vi "Teleop.vi"(10 "Match Info":T1={"Autonomous Elapsed Seconds"=0.0, "TeleOp Elapsed Seconds"=0.0, "Disabled Elapsed Seconds"=0.0, "Visited Autonomous"=FALSE, "Visited TeleOp"=FALSE, "Visited Disabled"=FALSE, "Autonomous Settings"={"Autonomous Style"=enum."Independent", "VI Refnum"=refnum}}, 11 "Call Context":T2) -> ()   [LabVIEW 2019]
doc: "This VI is called for each TeleOp packet received from the DS where the robot is not disabled. It is often used to read from the joysticks and update I/O or to update setpoints for timed control loops. It should complete and return within 20 milliseconds or it may miss DS packets."
uses:
  <vilib>/Rock Robotics/WPI/DriverStation/WPI_DriverStationDerivedRobotMode.ctl
  <vilib>/Rock Robotics/WPI/DriverStation/WPI_DriverStationMatch Info.ctl
  <vilib>/Rock Robotics/WPI/ThirdParty/JAS_Junk/TrajLib/Conv_Meters_Feet.vi
  <vilib>/Rock Robotics/WPI/ThirdParty/JAS_Junk/TrajLib/Conv_Radians_Deg.vi
  <vilib>/Rock Robotics/WPI/Utilities/WPI_GetSetVariantRefNum.vi
  <vilib>/Rock Robotics/Network Tables/NT Write Boolean Array.vi
  <vilib>/Rock Robotics/Network Tables/NT Write Numeric Array.vi
  Robot Global Data.vi
  <vilib>/Rock Robotics/Network Tables/NT Read Boolean.vi
  Secret_Control_Library_Protected/Secret_Control_Library_Protected.lvlib
  <vilib>/Rock Robotics/Network Tables/NT Read Number.vi
  <vilib>/Rock Robotics/WPI/ThirdParty/JAS_Junk/TrajLib/Trajectory_Library.lvlib
panel:
  out "Sample Slider 0":dbl(slide) scale=0.0..5.0
  out "Sample Boolean 1":bool
  out "Sample Boolean 0":bool
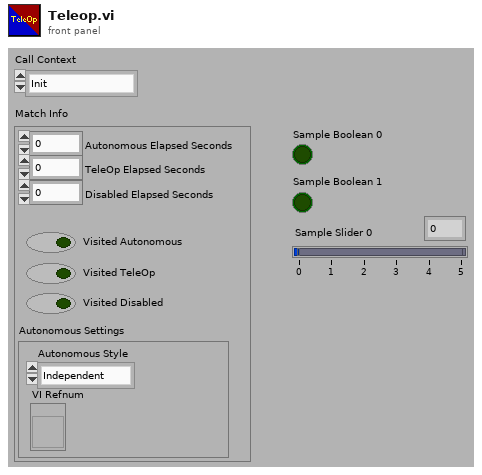
[diagram p1: front panel]
types:
  T1 = typedef "WPI_DriverStationMatch Info.ctl" = cluster{"Autonomous Elapsed Seconds":dbl, "TeleOp Elapsed Seconds":dbl, "Disabled Elapsed Seconds":dbl, "Visited Autonomous":bool, "Visited TeleOp":bool, "Visited Disabled":bool, "Autonomous Settings":cluster{"Autonomous Style":enum16{"Iterative", "Independent"}, "VI Refnum":refnum<vi>}}
  T2 = typedef "WPI_DriverStationDerivedRobotMode.ctl" = enum16{"Init", "Execute", "Stop"}
  T3 = typedef "WPI_JoystickDevRef.ctl" = cluster{"Device":T4}
  T4 = typedef "WPI_JoystickDeviceEnum.ctl" = enum16{"USB 0", "USB 1", "USB 2", "USB 3", "USB 4", "USB 5"}
  T5 = typedef "Trajectory_Library.lvlib/POSE2D.ctl" = cluster{"TRANSLATION":T6, "ROTATION":T7}
  T6 = typedef "Trajectory_Library.lvlib/TRANSLATION2D.ctl" = cluster{"X":dbl, "Y":dbl}
  T7 = typedef "Trajectory_Library.lvlib/ROTATION2D.ctl" = cluster{"VALUE":dbl, "COS":dbl, "SIN":dbl}
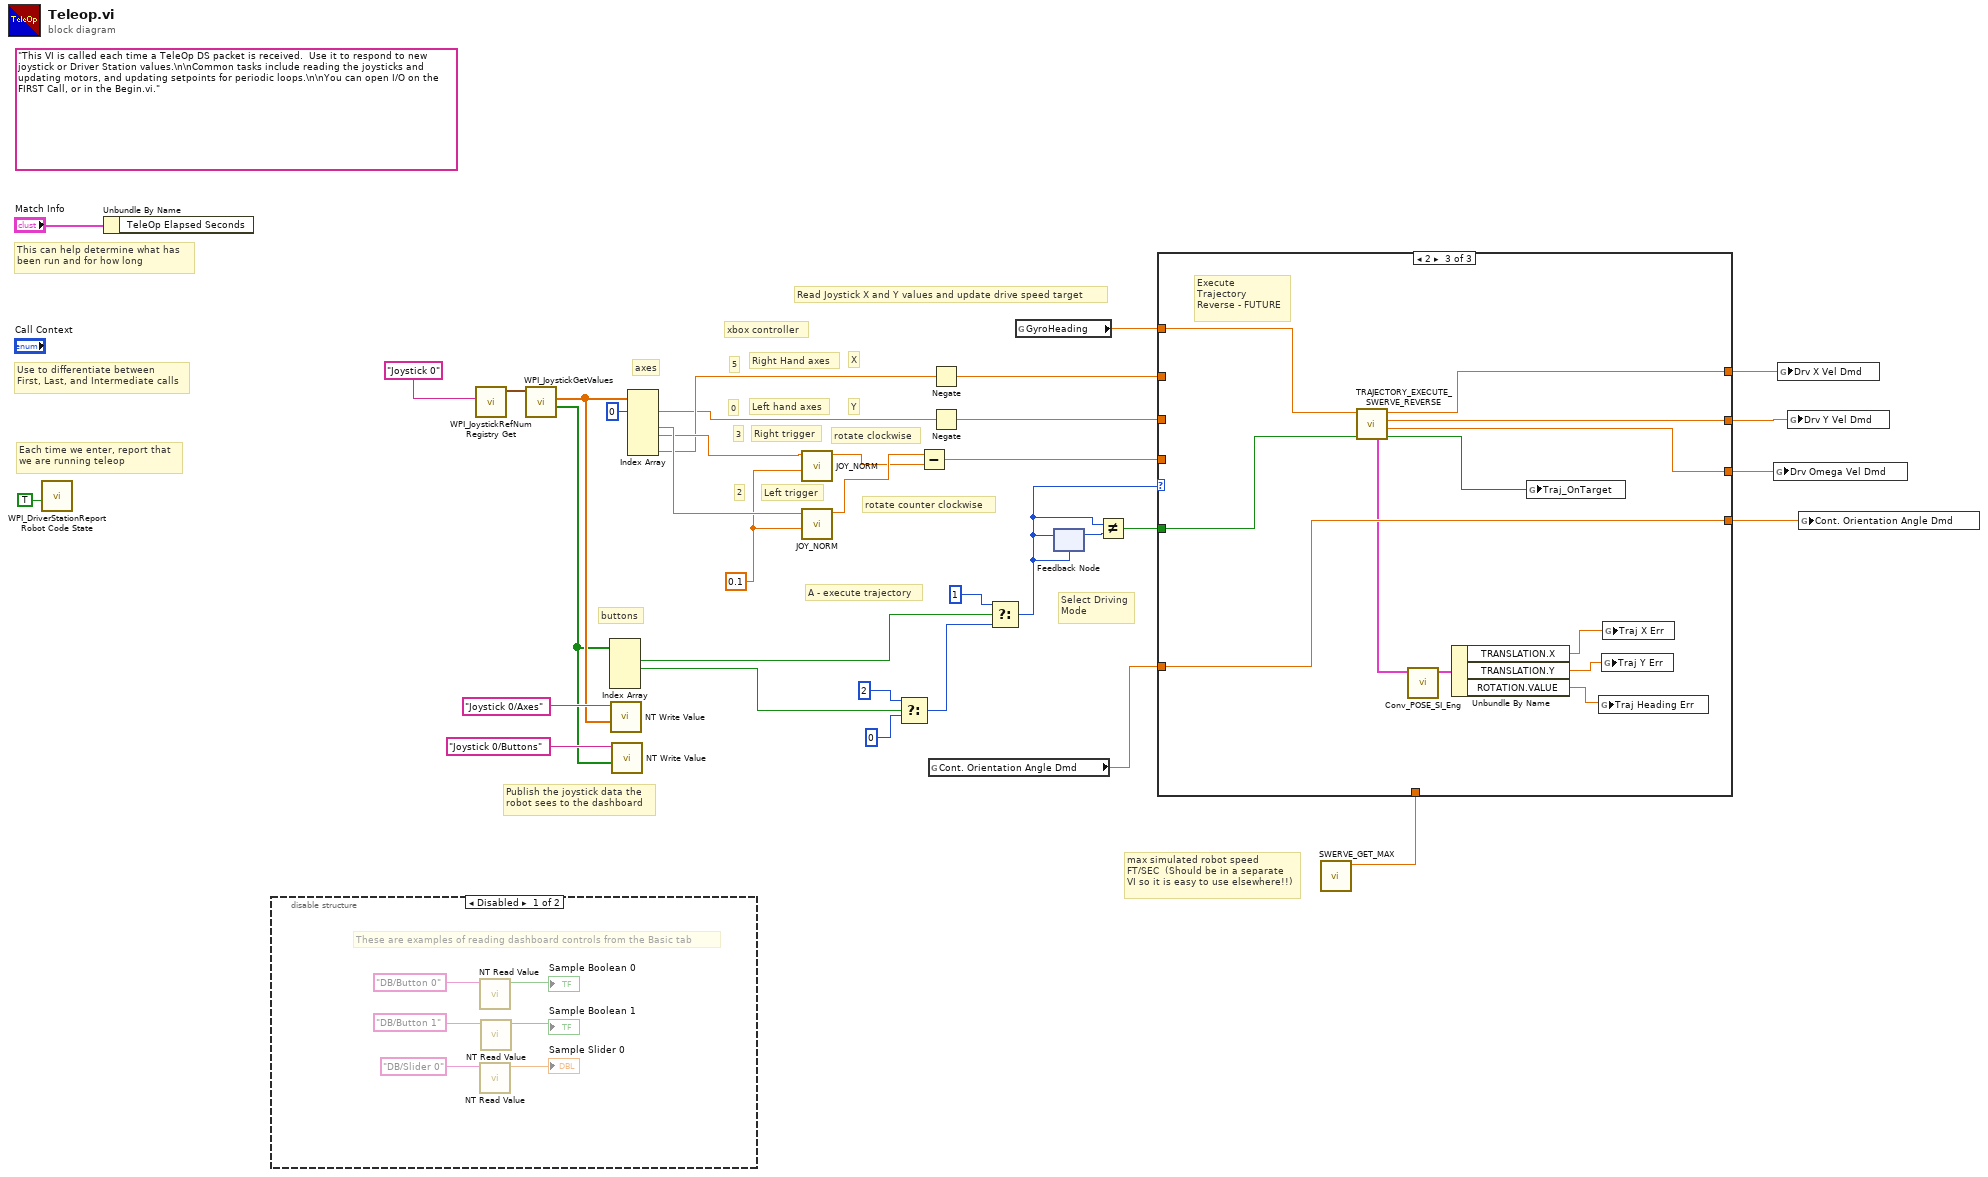
[diagram p0: block diagram]
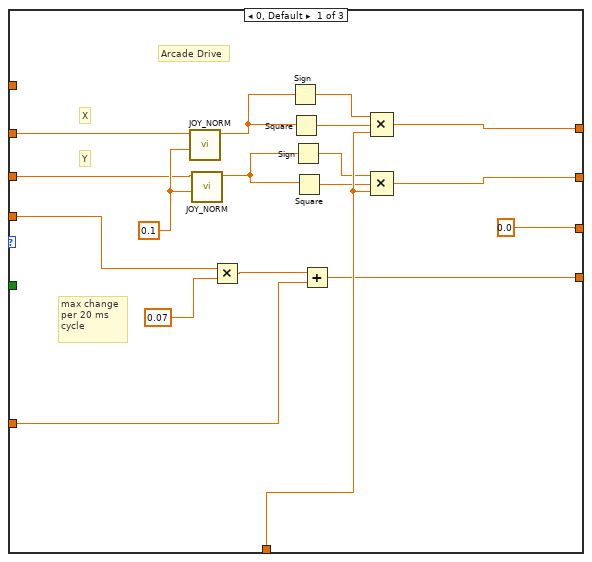
[diagram p2: hidden frame]
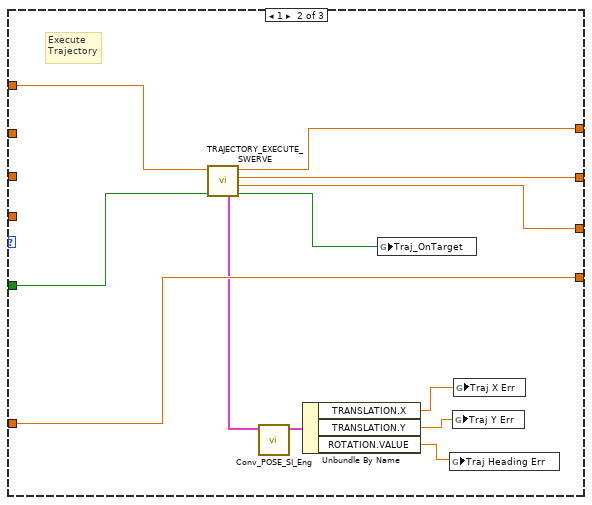
[diagram p3: hidden frame]
diagram:
  w13 = 0.1 ("Deadband")
  (unwired) "This VI is called each time a TeleOp DS packet is received.  Use it to respond to new joystick or Driver Station values.\n\nCommon tasks include reading the joysticks and updating motors, and updating setpoints for periodic loops.\n\nYou can open I/O on the FIRST Call, or in the Begin.vi."
  # "A - execute trajectory"
  # "xbox controller"
  # "Left trigger"
  # "rotate counter clockwise"
  # "2"
  # "Right trigger"
  # "rotate clockwise"
  # "3"
  # "Right Hand axes"
  # "5"
  # "0"
  # "Left hand axes"
  # "Y"
  # "X"
  # "Select Driving\nMode"
  # "buttons"
  # "axes"
  # "max simulated robot speed\nFT/SEC  (Should be in a separate\nVI so it is easy to use elsewhere!!)"
  # "Publish the joystick data the\nrobot sees to the dashboard"
  # "Each time we enter, report that\nwe are running teleop"
  # "Use to differentiate between\nFirst, Last, and Intermediate calls"
  # "This can help determine what has\nbeen run and for how long"
  # "Read Joystick X and Y values and update drive speed target"
  n1 = call <vilib>:"WPI_DriverStationReport Robot Code State.vi"("TeleOp"=TRUE ("Autonomous")) -> ()  [unwired: 10 in, 1 out]
  n2 = Unbundle By Name("Match Info") -> ()  [unwired: 1 out]
  n3 = disable-structure shown="Disabled" {
    frame Disabled {
      # "These are examples of reading dashboard controls from the Basic tab"
      n4 = call-poly <vilib>:"NT Read Value.vi"("Name"="DB/Button 0" ("refnum name")) -> ("Boolean"=→"Sample Boolean 0":bool)  [unwired: 9 in, 1 out]
      n5 = call-poly <vilib>:"NT Read Value.vi"("Name"="DB/Slider 0" ("refnum name")) -> ("Numeric"=→"Sample Slider 0":dbl)  [unwired: 9 in, 1 out]
      n6 = call-poly <vilib>:"NT Read Value.vi"("Name"="DB/Button 1" ("refnum name")) -> ("Boolean"=→"Sample Boolean 1":bool)  [unwired: 9 in, 1 out]
    }
    frame Enabled {
    }
  }
  n7 = call <vilib>:"WPI_JoystickRefNum Registry Get.vi"("refnum name"="Joystick 0") -> ("JoystickDevRef"=w33:T3)  [unwired: 1 in, 9 out]
  n8 = call <vilib>:"WPI_JoystickGetValues.vi"("JoystickDevRef"=w33) -> ("Buttons"=w26:bool[], "Axes"=w29:dbl[])  [unwired: 6 in, 3 out]
  n9 = Index Array(array=w26) -> (element #1=w24:bool, element #2=w2:bool)  [unwired: 4 in, 2 out]
  n10 = call-poly <vilib>:"NT Write Value.vi"("Numeric Array"=w29, "Name"="Joystick 0/Axes") -> ()  [unwired: 9 in, 1 out]
  n11 = call-poly <vilib>:"NT Write Value.vi"("Boolean Array"=w26, "Name"="Joystick 0/Buttons") -> ()  [unwired: 9 in, 1 out]
  n12 = Index Array(array=w29, index #1=0 ("index")) -> (element #1=w8:dbl, element #3=w15:dbl, element #4=w14:dbl, element #6=w9:dbl)  [unwired: 5 in, 2 out]
  n13 = call "JOY_NORM.vi"("Deadband"=w13, "Joy Input"=w14) -> ("Joy Output"=w5:dbl)  [unwired: 9 in]
  n14 = call "JOY_NORM.vi"("Deadband"=w13, "Joy Input"=w15) -> ("Joy Output"=w6:dbl)  [unwired: 9 in]
  n15 = Select(t=2, s=w2, f=0) -> (s? t:f=w1:i32)
  n16 = Subtract(x=w6, y=w5) -> (x-y=w12:dbl)
  n17 = global read "Robot Global Data.vi" "Cont. Orientation Angle Dmd"() -> (w18:dbl)
  n18 = Negate(x=w9) -> (-x=w10:dbl)
  n19 = Negate(x=w8) -> (-x=w7:dbl)
  n20 = Select(t=1, s=w24, f=w1) -> (s? t:f=w22:i32)
  n21 = global read "Robot Global Data.vi" "GyroHeading"() -> (w11:dbl)
  n22 = feedback-in #1(w22) -> ()
  n23 = feedback #1(w22) -> (w23:i32)
  n24 = Not Equal?(x=w22, y=w23) -> (x != y?=w21:bool)
  n25 = call "SWERVE_GET_MAX.vi"() -> ("Max Wheel Vel (Meter/Sec)"=w20:dbl)  [unwired: 10 in, 1 out]
  n26 = case shown="2" w22 {
    tunnel: w7 -> [w48 _ _]
    tunnel: [w58 w66 w78] -> w28
    tunnel: [w57 w65 w77] -> w27
    tunnel: w20 -> [w56 _ _]
    tunnel: w21 -> [_ w62 w74]
    tunnel: [w46 w67 w79] -> w19
    tunnel: w18 -> [w45 w67 w79]
    tunnel: [0.0 w64 w76] -> w17
    tunnel: w10 -> [w47 _ _]
    tunnel: w12 -> [w42 _ _]
    tunnel: w11 -> [_ w61 w73]
    frame 0, Default {
      w59 = 0.1 ("Deadband")
      # "max change\nper 20 ms\ncycle"
      # "Y"
      # "X"
      # "Arcade Drive"
      n27 = call "JOY_NORM.vi"("Deadband"=w59, "Joy Input"=w47) -> ("Joy Output"=w53:dbl)  [unwired: 9 in]
      n28 = call "JOY_NORM.vi"("Deadband"=w59, "Joy Input"=w48) -> ("Joy Output"=w50:dbl)  [unwired: 9 in]
      n29 = Multiply(x=w42, y=0.07) -> (x*y=w44:dbl)
      n30 = Sign(1:w53) -> (0:w54:dbl)
      n31 = Square(x=w53) -> (x^2=w55:dbl)
      n32 = Sign(1:w50) -> (0:w51:dbl)
      n33 = Square(x=w50) -> (x^2=w52:dbl)
      n34 = Add(x=w44, y=w45) -> (x+y=w46:dbl)
      n35 = Compound Arithmetic op=MULTIPLY(w54, w55, w56) -> (w58:dbl)
      n36 = Compound Arithmetic op=MULTIPLY(w51, w52, w56) -> (w57:dbl)
    }
    frame 1 {
      # "Execute\nTrajectory"
      n37 = call "TRAJECTORY_EXECUTE_SWERVE.vi"("Init"=w62, "Gyro Heading"=w61) -> ("AtReference"=w63:bool, "Omega Velocity Target"=w64:dbl, "Y Velocity Target"=w65:dbl, "X Velocoty Target"=w66:dbl, "Error Pose"=w60:T5)  [unwired: 5 in]
      n38 = call <vilib>:"Conv_POSE_SI_Eng.vi"("Err Pose in SI"=w60) -> ("Err Pose out ENG"=w71:T5)  [unwired: 10 in]
      n39 = Unbundle By Name(w71) -> ("TRANSLATION.X"=w70:dbl, "TRANSLATION.Y"=w69:dbl, "ROTATION.VALUE"=w68:dbl)
      n40 = global write "Robot Global Data.vi" "Traj_OnTarget"(w63) -> ()
      n41 = global write "Robot Global Data.vi" "Traj Heading Err"(w68) -> ()
      n42 = global write "Robot Global Data.vi" "Traj Y Err"(w69) -> ()
      n43 = global write "Robot Global Data.vi" "Traj X Err"(w70) -> ()
    }
    frame 2 {
      # "Execute\nTrajectory\nReverse - FUTURE"
      n44 = call "TRAJECTORY_EXECUTE_SWERVE_REVERSE.vi"("Init"=w74, "Gyro Heading"=w73) -> ("AtReference"=w75:bool, "Omega Velocity Target"=w76:dbl, "Y Velocity Target"=w77:dbl, "X Velocoty Target"=w78:dbl, "Error Pose"=w72:T5)  [unwired: 5 in]
      n45 = call <vilib>:"Conv_POSE_SI_Eng.vi"("Err Pose in SI"=w72) -> ("Err Pose out ENG"=w83:T5)  [unwired: 10 in]
      n46 = Unbundle By Name(w83) -> ("TRANSLATION.X"=w82:dbl, "TRANSLATION.Y"=w81:dbl, "ROTATION.VALUE"=w80:dbl)
      n47 = global write "Robot Global Data.vi" "Traj_OnTarget"(w75) -> ()
      n48 = global write "Robot Global Data.vi" "Traj Heading Err"(w80) -> ()
      n49 = global write "Robot Global Data.vi" "Traj Y Err"(w81) -> ()
      n50 = global write "Robot Global Data.vi" "Traj X Err"(w82) -> ()
    }
  }
  n51 = global write "Robot Global Data.vi" "Drv Omega Vel Dmd"(w17) -> ()
  n52 = global write "Robot Global Data.vi" "Drv X Vel Dmd"(w28) -> ()
  n53 = global write "Robot Global Data.vi" "Drv Y Vel Dmd"(w27) -> ()
  n54 = global write "Robot Global Data.vi" "Cont. Orientation Angle Dmd"(w19) -> ()
